vi "SP Coerce Limts to Valid Values.vi"(7 "Attribute Name (NI_ChannelName)":string="NI_ChannelName", 8 "error in (no error)":errorcluster, 9 "Units":T2, 10 "Limits":T4[](array[typedef]) {"Parameter"."Stimulus Port" min=1 step=1; "Parameter"."Response Port" min=1 step=1}, 11 "Results":waveform(dbl)[](array[waveform])) -> (0 "error out":errorcluster, 1 "Lower Limit Traces":cluster{"X":dbl[], "Y":dbl[]}[](array[cluster]), 2 "Upper Limit Traces":cluster{"X":dbl[], "Y":dbl[]}[](array[cluster]), 3 "dup Results":waveform(dbl)[](array[waveform]), 4 "Lower Limit Types":T3[](array[typedef]), 5 "Upper Limit Types":T3[](array[typedef]))   [LabVIEW 2011]
uses:
  TypeDefs/SP Limit.ctl
  TypeDefs/SP Parameter.ctl
  TypeDefs/SP Format.ctl
  TypeDefs/SP Limit Type.ctl
  TypeDefs/SP Limit Point.ctl
  Test Referential Limit.ctl
  TypeDefs/SP Frequency Units.ctl
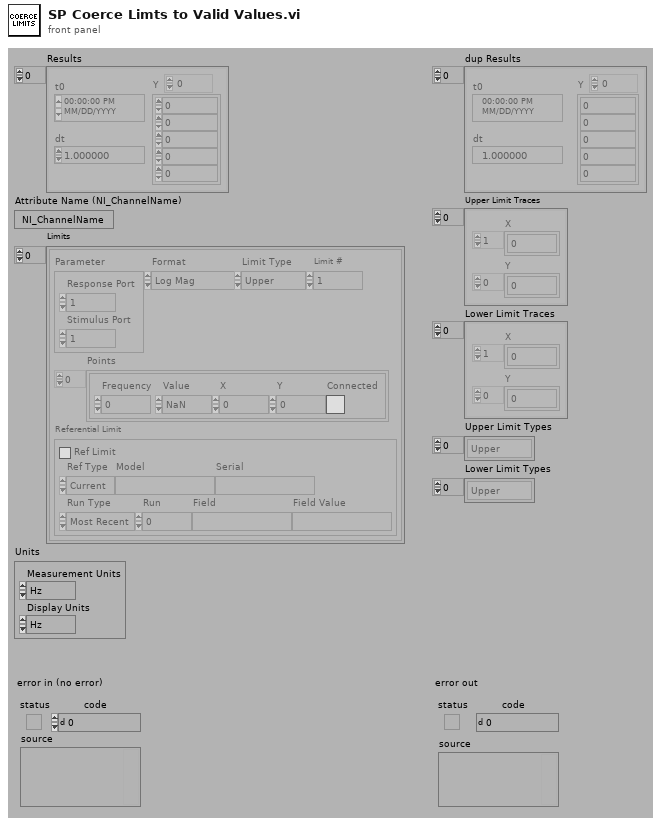
[diagram p1: front panel]
types:
  T1 = typedef "SP Frequency Units.ctl" = enum16{"Hz", "kHz", "MHz", "GHz", "Points"}
  T2 = cluster{"Measurement Units":T1, "Display Units":T1}
  T3 = typedef "SP Limit Type.ctl" = enum16{"Upper", "Lower", "Delta", "Filter", "Referential"}
  T4 = typedef "SP Limit.ctl" = cluster{"Parameter":T5, "Format":T6, "Limit Type":T3, "Points":T7[], "Referential Limit":T8, "Limit #":i8}
  T5 = typedef "SP Parameter.ctl" = cluster{"Stimulus Port":i8, "Response Port":i8}
  T6 = typedef "SP Format.ctl" = enum16{"Log Mag", "Lin Mag", "SWR", "Phase", "Expanded Phase", "Delay", "Insertion Loss", "Isolation", "Return Loss"}
  T7 = typedef "SP Limit Point.ctl" = cluster{"Frequency":dbl, "Value":dbl, "X":dbl, "Y":dbl, "Connected":bool}
  T8 = typedef "Test Referential Limit.ctl" = cluster{"Ref Limit":bool, "Ref Type":enum16{"Current", "Specify"}, "Model":string, "Serial":string, "Run Type":enum16{"Most Recent", "Run #", "Match Field"}, "Run":i32, "Field":string, "Field Value":string}
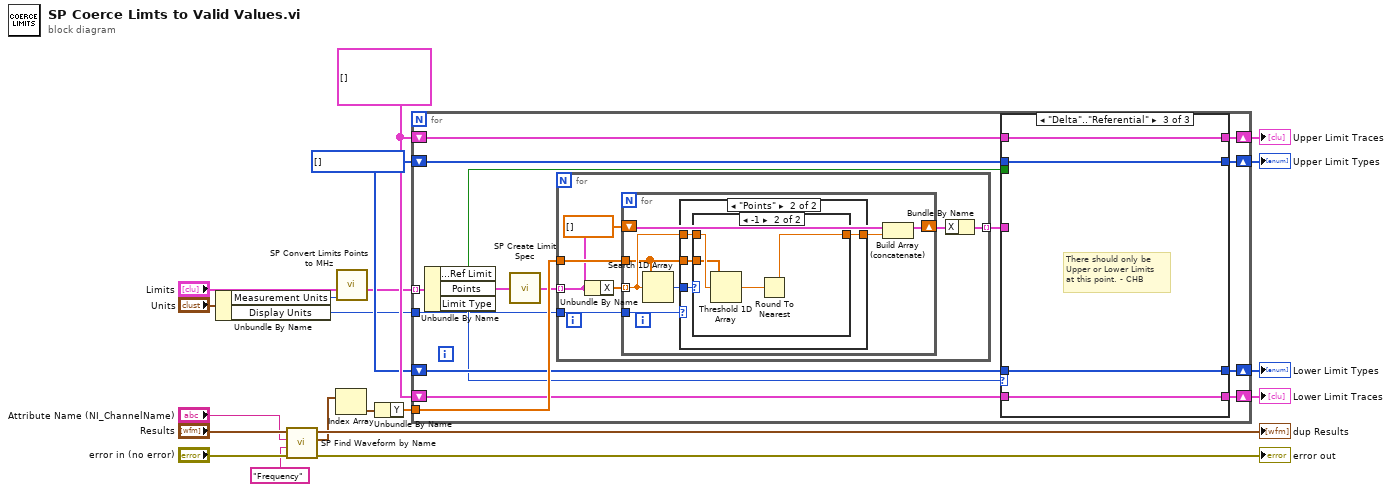
[diagram p0: block diagram]
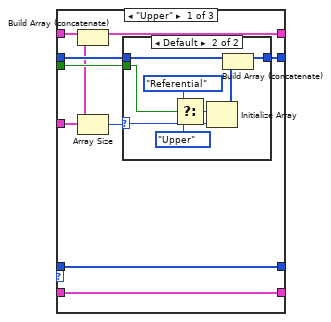
[diagram p2: hidden frame]
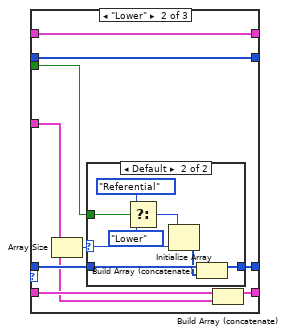
[diagram p4: hidden frame]
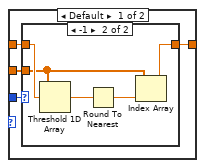
[diagram p6: hidden frame]
diagram:
  w8 = T3[] [] items=["Upper", "Lower", "Delta", "Filter", "Referential"] ("Upper Limit Traces")
  w11 = cluster{"X":dbl[], "Y":dbl[]}[] [] ("Upper Limit Traces")
  n1 = Unbundle By Name("Units") -> ("Measurement Units"=w2:T1, "Display Units"=w1:T1)
  n2 = call "SP Find Waveform by Name.vi"("error in (no error)"="error in (no error)", "Attribute Value (\"\")"="Frequency", "Attribute Name (NI_ChannelName)"="Attribute Name (NI_ChannelName)", "Results"="Results") -> ("error out"=→"error out":errorcluster, "Waveforms"=w10:waveform(dbl)[], "dup Results"=→"dup Results":waveform(dbl)[])  [unwired: 1 out]
  n3 = Index Array(array=w10) -> (element=w9:waveform(dbl))  [unwired: 1 in]
  n4 = call "SP Convert Limits Points to MHz.vi"("Units"=w2, "Limits In"="Limits") -> ("Limits Out"=w4:T4[])  [unwired: 5 out]
  n5 = Unbundle By Name(w9) -> ("Y"=w14:dbl[])
  n6 = for {
    tunnel: w4 -> [w36] mode=indexing
    tunnel: w14 -> [w35]
    shift-right: [w31] -> w12
    shift-left: w11 -> [w32]
    shift-right: [w29] -> w13
    shift-left: w11 -> [w30]
    shift-right: [w26] -> w7
    shift-left: w8 -> [w27]
    shift-right: [w25] -> w6
    shift-left: w8 -> [w24]
    tunnel: w1 -> [w21]
    n7 = Unbundle By Name(w36) -> ("Referential Limit.Ref Limit"=w23:bool, "Points"=w33:T7[], "Limit Type"=w22:T3)
    n8 = call "SP Create Limit Spec.vi"("Limit"=w33) -> ("Limit Traces"=w34:cluster{"X":dbl[], "Y":dbl[]}[])  [unwired: 1 in, 3 out]
    n9 = for {
      tunnel: w34 -> [w80] mode=indexing
      tunnel: w35 -> [w82]
      tunnel: [w79] -> w28 mode=indexing
      tunnel: w21 -> [w77]
      n10 = Unbundle By Name(w80) -> ("X"=w83:dbl[])
      n11 = for {
        tunnel: w83 -> [w89] mode=indexing
        tunnel: w82 -> [w86]
        shift-right: [w85] -> w78
        shift-left: dbl[] [] -> [w87]
        tunnel: w77 -> [w84]
        n12 = Search 1D Array(1D array=w86, element=w89) -> (index of element=w90:i32)  [unwired: 1 out]
        n13 = case shown="\"Points\"" w84 {
          tunnel: w90 -> [w94 w104]
          tunnel: w89 -> [w93 w103]
          tunnel: [w92 w102] -> w88
          tunnel: w86 -> [w91 w101]
          frame Default {
            n14 = case shown="-1" w94 {
              tunnel: w93 -> [w95 w100]
              tunnel: [w95 w98] -> w92
              tunnel: w91 -> [_ w99]
              frame Default {
              }
              frame -1 {
                n15 = Threshold 1D Array(2:w100, 3:w99) -> (0:w97:dbl)  [unwired: 1 out]
                n16 = Round To Nearest(number=w97) -> (nearest integer value=w96:dbl)
                n17 = Index Array(array=w99, index=w96) -> (element=w98:dbl)
              }
            }
          }
          frame "Points" {
            n18 = case shown="-1" w104 {
              selector: w104 -> [w105 _]
              tunnel: w103 -> [_ w109]
              tunnel: [w105 w106] -> w102
              tunnel: w101 -> [_ w108]
              frame Default {
              }
              frame -1 {
                n19 = Threshold 1D Array(2:w109, 3:w108) -> (0:w107:dbl)  [unwired: 1 out]
                n20 = Round To Nearest(number=w107) -> (nearest integer value=w106:dbl)
              }
            }
          }
        }
        n21 = Build Array (concatenate)(w87, w88) -> (w85:dbl[])
      }
      n22 = Bundle By Name(cluster=w80, "X"=w78) -> (w79:cluster{"X":dbl[], "Y":dbl[]})
    }
    n23 = case shown="\"Delta\"..\"Referential\"" w22 {
      tunnel: w32 -> [w45 w57 w76]
      tunnel: [w44 w57 w76] -> w31
      tunnel: w30 -> [w37 w63 w74]
      tunnel: [w37 w62 w74] -> w29
      tunnel: w28 -> [w39 w58 _]
      tunnel: w27 -> [w42 w56 w75]
      tunnel: [w41 w56 w75] -> w26
      tunnel: [w38 w60 w73] -> w25
      tunnel: w24 -> [w38 w59 w73]
      tunnel: w23 -> [w40 w55 _]
      frame "Upper" {
        n24 = Build Array (concatenate)(w45, w39) -> (w44:cluster{"X":dbl[], "Y":dbl[]}[])
        n25 = Array Size(array=w39) -> (size(s)=w43:i32)
        n26 = case shown="Default" w43 {
          selector: w43 -> [_ w51]
          tunnel: w42 -> [w46 w54]
          tunnel: [w46 w53] -> w41
          tunnel: w40 -> [_ w49]
          frame 0 {
          }
          frame Default {
            n27 = Select(t=SP_Limit_Type."Referential", s=w49, f=SP_Limit_Type."Upper") -> (s? t:f=w50:T3)
            n28 = Initialize Array(w50, w51) -> (w52:T3[])
            n29 = Build Array (concatenate)(w54, w52) -> (w53:T3[])
          }
        }
      }
      frame "Lower" {
        n30 = Array Size(array=w58) -> (size(s)=w61:i32)
        n31 = case shown="Default" w61 {
          selector: w61 -> [_ w70]
          tunnel: w59 -> [w64 w72]
          tunnel: [w64 w71] -> w60
          tunnel: w55 -> [_ w65]
          frame 0 {
          }
          frame Default {
            n32 = Select(t=SP_Limit_Type."Referential", s=w65, f=SP_Limit_Type."Lower") -> (s? t:f=w66:T3)
            n33 = Initialize Array(w66, w70) -> (w69:T3[])
            n34 = Build Array (concatenate)(w72, w69) -> (w71:T3[])
          }
        }
        n35 = Build Array (concatenate)(w63, w58) -> (w62:cluster{"X":dbl[], "Y":dbl[]}[])
      }
      frame "Delta".."Referential" {
        # "There should only be\nUpper or Lower Limits\nat this point. - CHB"
      }
    }
  }
  "Lower Limit Traces" <- w13
  "Upper Limit Traces" <- w12
  "Upper Limit Types" <- w7
  "Lower Limit Types" <- w6
